vi "_Read Spectrum.vi"(0 "file path":path, 3 "AcqMethod":T1[](array[typedef]) {"ScanType" format="%#.6g"; "Mass Range"."Res" items=["High/High", "Medium/Medium", "Low/Low", "High/Medium", "High/Low", "Medium/High", "Medium/Low", "Low/High", "Low/Medium"]}, 5 "Scan# (1-based)":i32=1, 7 "Expt# (1-based)":i32=1, 9 "MR# (1-based)":i32=1, 11 "error in (no error)":errorcluster) -> (1 "Expt# Out":i32=1, 2 "MR# Out":i32=1, 4 "Data":T6, 6 "Scan# out":i32=1, 10 "Version":i32, 12 "raw data":i32[](array[numeric]), 15 "error out":errorcluster)   [LabVIEW 2012]
uses:
  Type/_Data.ctl
  Type/_XML Expt.ctl
  Type/_XML Lens.ctl
  Type/_Mass Range Property.ctl
  Type/_Mass Range Parameters.ctl
  Type/_RT Res Type.ctl
panel:
  out "Index Array":i64[][](array[numeric])
  out "Steps":i32[][](array[numeric])
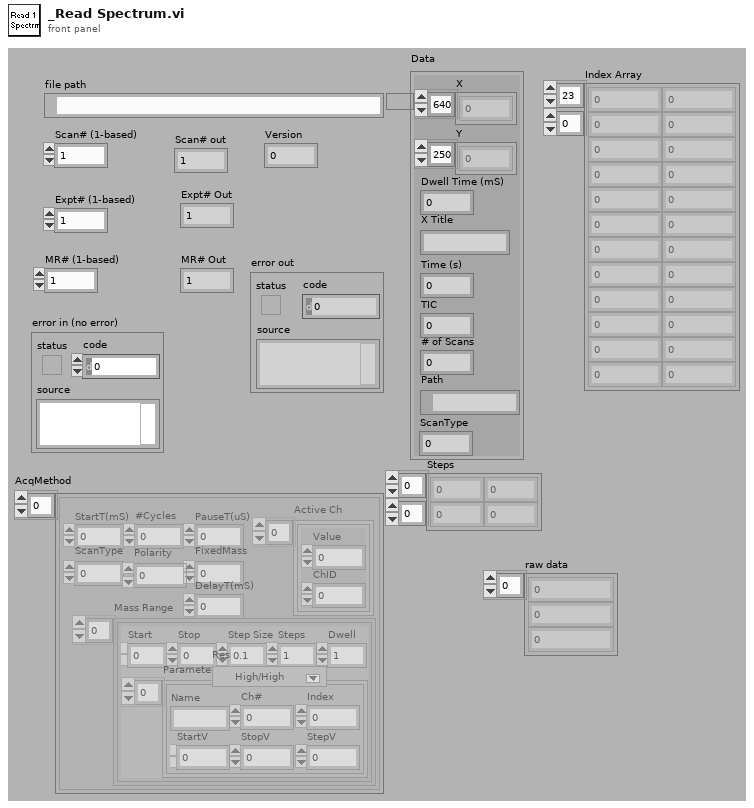
[diagram p1: front panel]
types:
  T1 = typedef "_XML Expt.ctl" = cluster{"StartT(mS)":i32, "#Cycles":i32, "PauseT(uS)":i32, "ScanType":i32, "Polarity":u8, "FixedMass":dbl, "DelayT(mS)":i32, "Active Ch":T2[], "Mass Range":T3[]}
  T2 = typedef "_XML Lens.ctl" = cluster{"Value":dbl, "ChID":u8}
  T3 = typedef "_Mass Range Property.ctl" = cluster{"Start":dbl, "Stop":dbl, "Step Size":dbl, "Steps":i32, "Dwell":dbl, "Parameters":T4[], "Res":T5}
  T4 = typedef "_Mass Range Parameters.ctl" = cluster{"Name":string, "Ch#":u8, "StartV":dbl, "StopV":dbl, "StepV":dbl, "Index":u8}
  T5 = typedef "_RT Res Type.ctl" = u16
  T6 = typedef "_Data.ctl" = cluster{"X":dbl[], "Y":dbl[], "Dwell Time (mS)":dbl, "X Title":string, "Time (s)":dbl, "TIC":u32, "# of Scans":i32, "Path":path, "ScanType":i32}
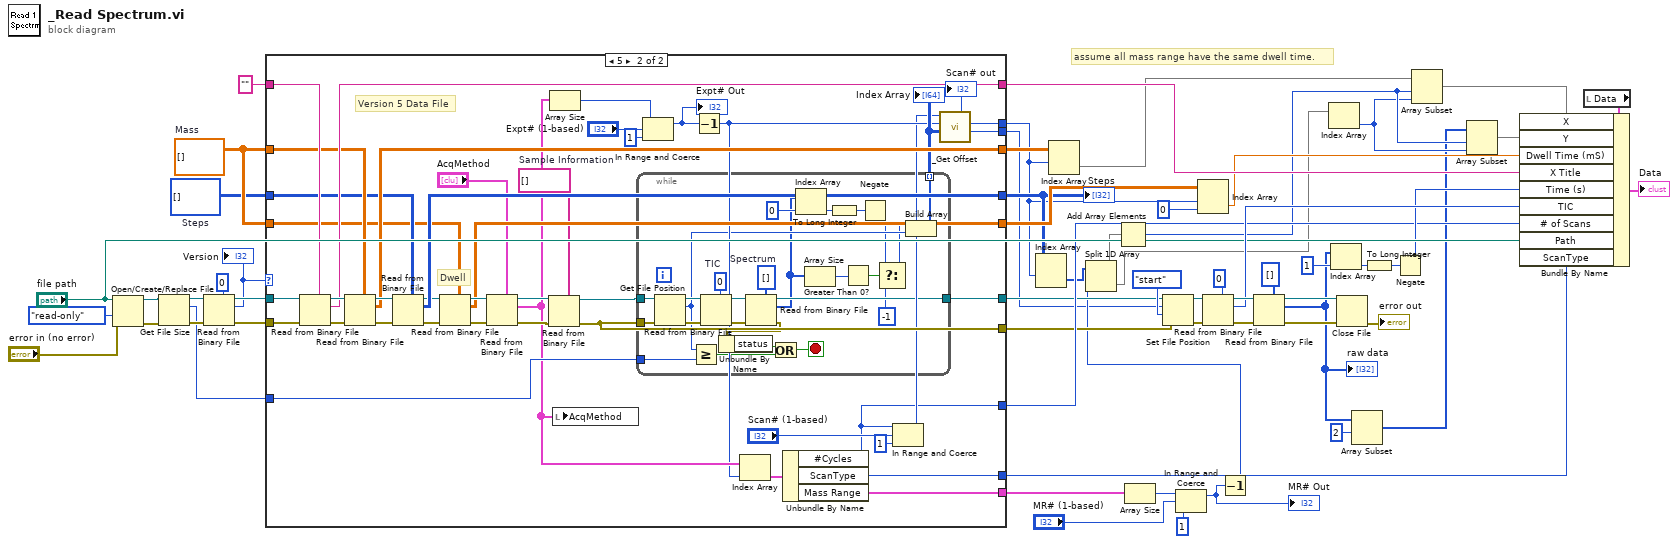
[diagram p0: block diagram]
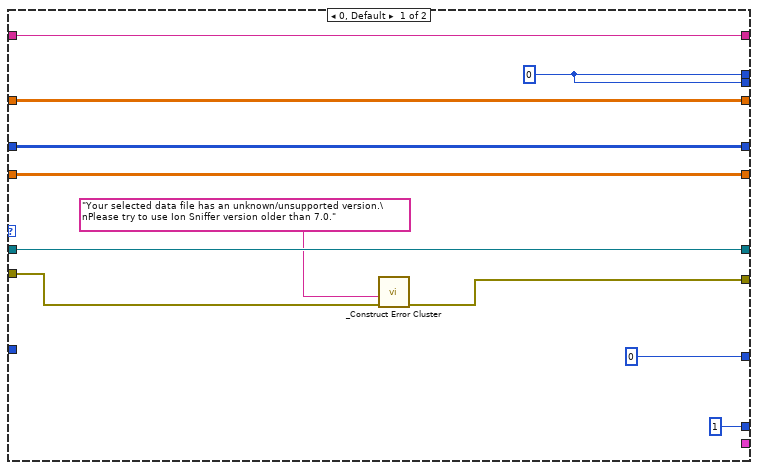
[diagram p2: hidden frame]
diagram:
  w25 = i32[][] []  # Steps
  w26 = dbl[][] []  # Mass
  # "assume all mass range have the same dwell time."
  n1 = Open/Create/Replace File(file path (use dialog)="file path", error in="error in (no error)", access (0:read/write)=enum16{"read/write", "read-only", "write-only"}."read-only") -> (refnum out=w50:refnum<file>, error out=w49:errorcluster)  [unwired: 4 out]
  n2 = Get File Size ("EOF")(file=w50, error in=w49) -> (refnum out=w38:refnum<file>, size (in bytes)=w34:i64, 0:w37:errorcluster)
  n3 = Read from Binary File(5:0 ("pos offset (0)"), 8:w37, 11:w38) -> (0:w35:errorcluster, 2:w23:i32, 3:w36:refnum<file>)  [unwired: 4 out]
  "Version" <- w23
  n4 = case shown="5" w23 {
    tunnel: w35 -> [w71 w112]
    tunnel: w36 -> [w72 w111]
    tunnel: [w66 w108] -> w27
    tunnel: [w67 w106] -> w31
    tunnel: [0 w73] -> w33
    tunnel: [w72 w96] -> w22
    tunnel: [w69 w92] -> w21
    tunnel: w34 -> [_ w95]
    tunnel: [w64 w107] -> w13
    tunnel: "" -> [w67 w105]
    tunnel: w26 -> [w66 w104]
    tunnel: w25 -> [w64 w103]
    tunnel: w26 -> [w65 w98]
    tunnel: [w65 w97] -> w29
    tunnel: [w62 w77] -> w12
    tunnel: [1 ("ScanType") w84] -> w18
    tunnel: [_ w82] -> w17
    tunnel: [w62 w75] -> w2
    frame 0, Default {
      w62 = 0 ("lower limit")
      n5 = call "_Construct Error Cluster.vi"("error in"=w71, "reason"="Your selected data file has an unknown/unsupported version.\nPlease try to use Ion Sniffer version older than 7.0.") -> ("error out"=w69:errorcluster)  [unwired: 2 in, 3 out]
    }
    frame 5 {
      w90 = string[] []  # Sample Information
      # "Dwell"
      # "Version 5 Data File"
      n6 = Read from Binary File(5:w105, 8:w112, 11:w111) -> (0:w114:errorcluster, 2:w106:string, 3:w110:refnum<file>)  [unwired: 4 out]
      n7 = Read from Binary File(5:w104, 8:w114, 11:w110) -> (0:w113:errorcluster, 2:w108:dbl[][], 3:w109:refnum<file>)  [unwired: 4 out]
      n8 = Read from Binary File(5:w103, 8:w113, 11:w109) -> (0:w100:errorcluster, 2:w107:i32[][], 3:w101:refnum<file>)  [unwired: 4 out]
      n9 = Read from Binary File(5:w98, 8:w100, 11:w101) -> (0:w102:errorcluster, 2:w97:dbl[][], 3:w99:refnum<file>)  [unwired: 4 out]
      n10 = Read from Binary File(5:"AcqMethod", 8:w102, 11:w99) -> (0:w91:errorcluster, 2:w83:T1[], 3:w94:refnum<file>)  [unwired: 4 out]
      n11 = Read from Binary File(5:w90, 8:w91, 11:w94) -> (0:w92:errorcluster, 3:w93:refnum<file>)  [unwired: 5 out]
      n12 = Array Size(array=w83) -> (size(s)=w86:i32)
      n13 = local write "AcqMethod"(w83) -> ()
      n14 = while {
        tunnel: w93 -> [w139]
        tunnel: w92 -> [w138]
        tunnel: [w136] -> w96
        tunnel: w95 -> [w135]
        tunnel: [w121] -> w78 mode=indexing
        stop <- w132 stop-if-true
        w127 = u32 0  # TIC
        w137 = u32[] []  # Spectrum
        n15 = Get File Position(4:w138, 7:w139) -> (0:w128:errorcluster, 2:w122:i64, 3:w130:refnum<file>)
        n16 = Greater Or Equal?(x=w122, y=w135) -> (x >= y?=w133:bool)
        n17 = Read from Binary File(5:w127, 8:w128, 11:w130) -> (0:w131:errorcluster, 3:w129:refnum<file>)  [unwired: 5 out]
        n18 = Read from Binary File(5:w137, 8:w131, 11:w129) -> (0:w126:errorcluster, 2:w120:u32[], 3:w136:refnum<file>)  [unwired: 4 out]
        n19 = Unbundle By Name(w126) -> ("status"=w134:bool)
        n20 = Or(x=w134, y=w133) -> (x .or. y?=w132:bool)
        n21 = Index Array(array=w120, index=0) -> (element=w124:u32)
        n22 = Array Size(array=w120) -> (size(s)=w119:i32)
        n23 = To Long Integer(number=w124) -> (32bit integer=w125:i32)
        n24 = Greater Than 0?(x=w119) -> (x > 0?=w118:bool)
        n25 = Negate(x=w125) -> (-x=w117:i32)
        n26 = Select(t=w117, s=w118, f=-1) -> (s? t:f=w115:i32)
        n27 = Build Array(w115, w122) -> (w121:i64[])
      }
      "Index Array" <- w78
      n28 = In Range and Coerce(upper limit=w86, x="Expt# (1-based)", lower limit=1) -> (coerced(x)=w81:i32)  [unwired: 1 out]
      "Expt# Out" <- w81
      n29 = Decrement(x=w81) -> (x-1=w77:i32)
      n30 = Index Array(array=w83, index=w77) -> (element=w85:T1)
      n31 = Unbundle By Name(w85) -> ("#Cycles"=w73:i32, "ScanType"=w84:i32, "Mass Range"=w82:T3[])
      n32 = In Range and Coerce(upper limit=w73, x="Scan# (1-based)", lower limit=1) -> (coerced(x)=w76:i32)  [unwired: 1 out]
      n33 = call "_Get Offset.vi"("Index Array"=w78, "Expt# (0-based)"=w77, "Scan# (1-based)"=w76) -> ("Offset"=w75:i64, "Scan# out"=→"Scan# out":i32)  [unwired: 3 out]
    }
  }
  "Steps" <- w13
  n34 = Index Array(array=w13, index (row)=w12) -> (element=w11:i32[])  [unwired: 1 in]
  n35 = Index Array(array=w27, index (row)=w12) -> (element=w20:dbl[])  [unwired: 1 in]
  n36 = Array Size(array=w17) -> (size(s)=w15:i32)
  n37 = Set File Position(offset (in bytes) (0)=w2, refnum=w22, from (0:start)=enum16{"start", "end", "current"}."start" ("pos mode (0:2)"), error in=w21) -> (refnum out=w47:refnum<file>, error out=w46:errorcluster)
  n38 = In Range and Coerce(upper limit=w15, x="MR# (1-based)", lower limit=1) -> (coerced(x)=w10:i32)  [unwired: 1 out]
  "MR# Out" <- w10
  n39 = Index Array(array=w29, index (row)=w12, index (col)=0 ("index (row)")) -> (element=w28:dbl)
  n40 = Read from Binary File(5:u32 0, 8:w46, 11:w47) -> (0:w58:errorcluster, 2:w53:u32, 3:w59:refnum<file>)  [unwired: 4 out]
  n41 = Decrement(x=w10) -> (x-1=w9:i32)
  n42 = Split 1D Array(array=w11, index=w9) -> (first subarray=w8:i32[], second subarray=w7:i32[])
  n43 = Add Array Elements(numeric array=w8) -> (sum=w6:i32)
  n44 = Read from Binary File(5:u32[] [] ("Spectrum"), 8:w58, 11:w59) -> (0:w56:errorcluster, 2:w1:u32[], 3:w57:refnum<file>)  [unwired: 4 out]
  "raw data" <- w1
  n45 = Index Array(array=w7) -> (element=w5:i32)  [unwired: 1 in]
  n46 = Index Array(array=w1, index=1) -> (element=w44:u32)
  n47 = Close File(refnum=w57, error in=w56) -> (error out=→"error out":errorcluster)  [unwired: 1 out]
  n48 = Array Subset(array=w1, index=2) -> (w3:u32[])  [unwired: 1 in]
  n49 = To Long Integer(number=w44) -> (32bit integer=w42:i32)
  n50 = Negate(x=w42) -> (-x=w41:i32)
  n51 = Array Subset(array=w20, index=w6, length=w5) -> (w19:dbl[])
  n52 = Array Subset(array=w3, index=w6, length=w5) -> (w4:u32[])
  n53 = local read "Data"() -> (w54:T6)
  n54 = Bundle By Name(cluster=w54, "X"=w19, "Y"=w4, "Dwell Time (mS)"=w28, "X Title"=w31, "Time (s)"=w41, "TIC"=w53, "# of Scans"=w33, "Path"="file path", "ScanType"=w18) -> (→"Data":T6)
